vi "HallOfFame.vi"(8 "error in":errorcluster, 11 "class data in":refnum<class "Game.lvclass">) -> (0 "error out":errorcluster, 3 "class data out":refnum<class "Game.lvclass">)   [LabVIEW 2010, in "Labricks.lvlib" / "Game.lvclass"]
uses:
  Game.lvclass
  <vilib>/Utility/miscctls.llb/LV3DPointTypeDef.ctl
  Game.lvclass/Game.ctl
  Text_class/Text.lvclass
  Text_class/properties/Text/SetText.vi
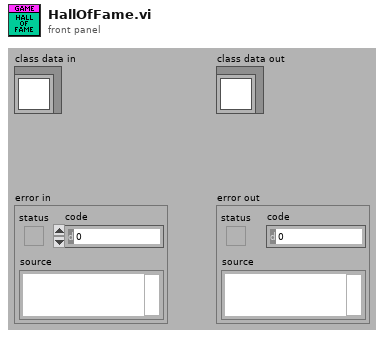
[diagram p1: front panel]
types:
  T1 = typedef "LV3DPointTypeDef.ctl" = cluster{"X":sgl, "Y":sgl, "Z":sgl}
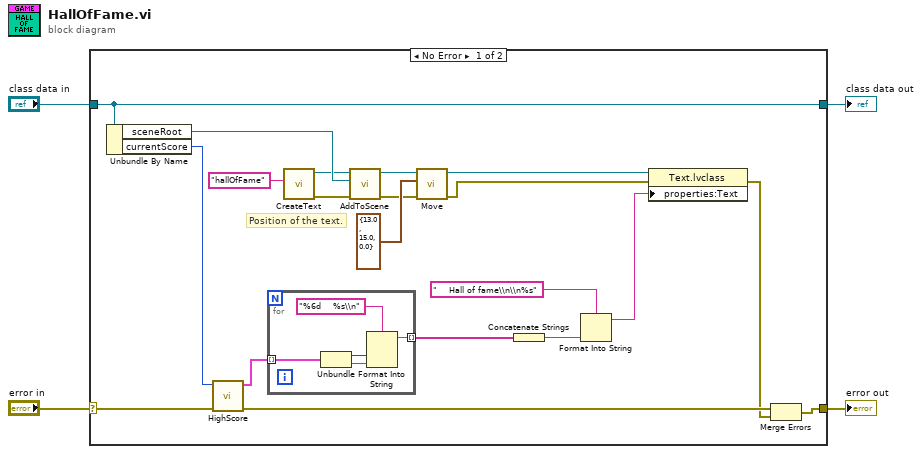
[diagram p0: block diagram]
diagram:
  n1 = case shown="No Error" "error in" {
    selector: "error in" -> [w18 w31]
    tunnel: [w13 w31] -> w4
    tunnel: "class data in" -> [w17 w30]
    tunnel: [w17 w30] -> w1
    frame No Error {
      # "Position of the text."
      n2 = Unbundle By Name(w17) -> ("sceneRoot"=w24:refnum<class "SceneRoot.lvclass">, "currentScore"=w19:i32)
      n3 = call "HighScore.vi"("error in"=w18, "score in"=w19) -> ("error out"=w20:errorcluster, "hallOfFame out"=w6:cluster{"score":i32, "name":string}[])  [unwired: 8 in]
      n4 = for {
        tunnel: w6 -> [w29] mode=indexing
        tunnel: [w25] -> w7 mode=indexing
        n5 = Unbundle(w29) -> ("score"=w28:i32, "name"=w27:string)
        n6 = Format Into String(format string="%6d    %s\\n", w28, w27) -> (resulting string=w25:string)  [unwired: 2 in, 1 out]
      }
      n7 = call "CreateText.vi"("objName in"="hallOfFame") -> ("error out"=w16:errorcluster, "class data out"=w23:refnum<class "Text.lvclass">)  [unwired: 9 in]
      n8 = call-dynamic "AddToScene.vi"("error in (no error)"=w16, "sceneRoot in"=w24, "class data in"=w23) -> ("error out"=w14:errorcluster, "class data out"=w15:refnum<class "Text.lvclass">)  [unwired: 7 in]
      n9 = call-dynamic "Move.vi"("error in (no error)"=w14, "targetCoords in"=T1 {"X"=13.0, "Y"=15.0, "Z"=0.0}, "class data in"=w15) -> ("error out"=w12:errorcluster, "class data out"=w11:refnum<class "Text.lvclass">)  [unwired: 7 in]
      n10 = Concatenate Strings(w7) -> (w8:string)
      n11 = Format Into String(format string="    Hall of fame\\n\\n%s", w8) -> (resulting string=w5:string)  [unwired: 2 in, 1 out]
      n12 = property class="Text.lvclass"(reference=w11, error in=w12, "properties:Text"=w5) -> (error out=w10:errorcluster)  [unwired: 1 out]
      n13 = Merge Errors(w20, w10) -> (w13:errorcluster)
    }
    frame Error {
    }
  }
  "error out" <- w4
  "class data out" <- w1
